vi "AnalogChannelToInputChannel.vi"(8 "error in (no error)":errorcluster, 10 "Optical Channel In":i32=1 min=1 max=4 step=1, 11 "System no.":i32=1 min=1 max=4 step=1) -> (0 "error out":errorcluster, 2 "Input Channel Out":i32=1 min=1 max=4 step=1)   [LabVIEW 2023]
doc: "Reads out the number of sensor channels and adds the analog input channel (the one that can be read out with TAV?).\nThe corresponding input channel is returned.\n\nThis means for example: The controller has 18 input channels with 14 sensor channels. The first analog input channel will then be returned as input channel 15."
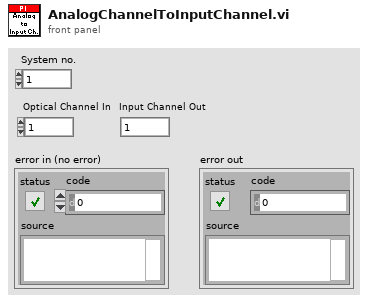
[diagram p1: front panel]
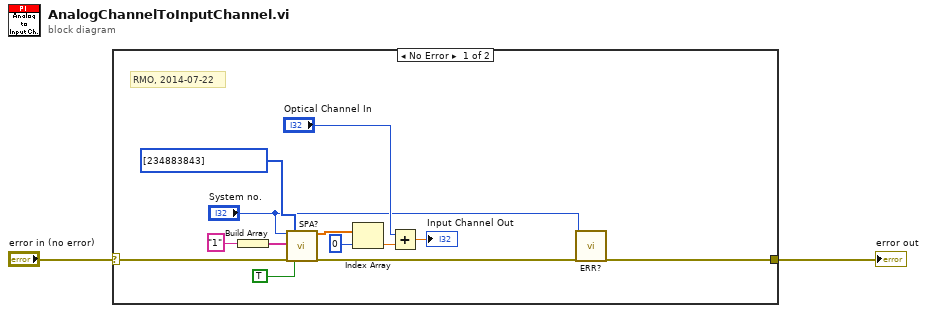
[diagram p0: block diagram]
diagram:
  n1 = case shown="No Error" "error in (no error)" {
    selector: "error in (no error)" -> [w13 w16]
    tunnel: [w5 w16] -> w2
    frame No Error {
      # "RMO, 2014-07-22"
      n2 = Build Array("1") -> (w14:string[])
      n3 = call "SPA?.vi"("System no."="System no.", "Axes to query"=w14, "error in"=w13, "Parameter no. (hex)"=u32[] [234883843], "Parameter no. format \n(Decimal: FALSE)"=TRUE ("Parameter no. format \n(Decimal: FALSE)")) -> ("Parameter value"=w9:dbl[], "error out"=w4:errorcluster)  [unwired: 9 in, 4 out]
      n4 = Index Array(array=w9, index=0) -> (element=w6:dbl)
      n5 = Add(x="Optical Channel In", y=w6) -> (x+y=→"Input Channel Out":dbl)
      n6 = call "ERR?.vi"("System no."="System no.", "error in"=w4) -> ("error out"=w5:errorcluster)  [unwired: 16 in, 1 out]
    }
    frame Error {
    }
  }
  "error out" <- w2
